vi "SL TAGS Reset Server Update Count.vi"(8 "error in (no error)":errorcluster, 11 "EEISysLink in":refnum<class "EEISysLink.lvclass">) -> (0 "error out":errorcluster, 3 "EEISysLink out":refnum<class "EEISysLink.lvclass">)   [LabVIEW 2017, in "EEISysLink.lvclass"]
doc: "Reset the internal count of number of tags that have been updated to the server. \n\nJames Tillett\nEndeavor Engineering Inc.\nwww.endeavoreng.com"
uses:
  EEISysLink.lvclass
  EEISysLink.lvclass/EEISysLink.ctl
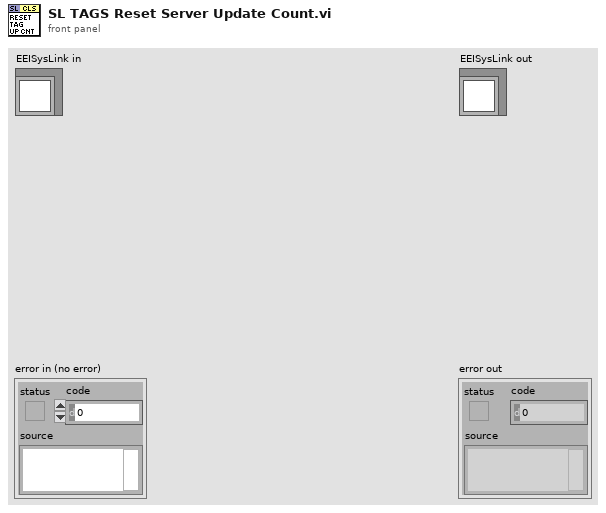
[diagram p1: front panel]
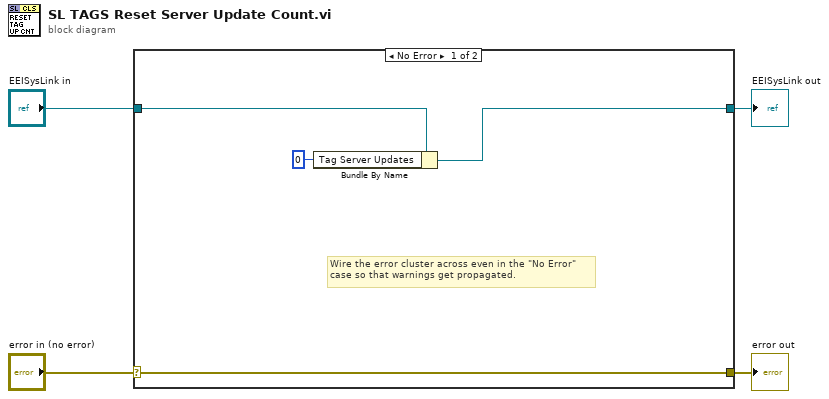
[diagram p0: block diagram]
diagram:
  n1 = case shown="No Error" "error in (no error)" {
    selector: "error in (no error)" -> [w8 w10]
    tunnel: [w8 w10] -> w3
    tunnel: [w5 w9] -> w1
    tunnel: "EEISysLink in" -> [w6 w9]
    frame No Error {
      # "Wire the error cluster across even in the \"No Error\"\ncase so that warnings get propagated."
      n2 = Bundle By Name(cluster=w6, "Tag Server Updates"=0) -> (w5:refnum<class "EEISysLink.lvclass">)
    }
    frame Error {
    }
  }
  "error out" <- w3
  "EEISysLink out" <- w1
